vi "Process Methods.vi"(8 "error in (no error)":errorcluster {"code" format="Error %.0f"}, 10 "UIs":refnum<class "GUI Documentation.lvclass">[](array[class]), 11 "VIDoc Printer In":refnum<class "VIDoc Printer.lvclass">) -> (0 "error out":errorcluster {"code" format="Error %.0f"}, 3 "VIDoc Printer Out":refnum<class "VIDoc Printer.lvclass">)   [LabVIEW 2023, in "VIDoc Printer.lvlib" / "VIDoc Printer.lvclass"]
uses:
  VIDoc Printer.lvclass
  VIDoc Printer.lvclass/VIDoc Printer.ctl
  Parsing/GUI Documentation/GUI Documentation.lvclass
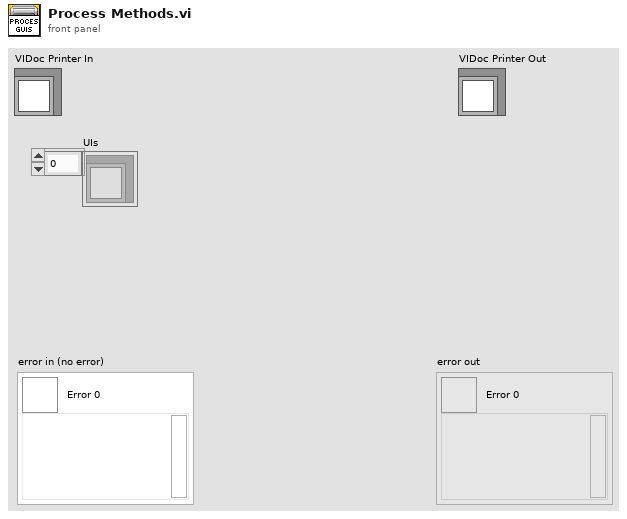
[diagram p1: front panel]
types:
  T1 = typedef "VIDoc Printer.lvlib/VIDoc Printer.lvclass/Process VI Enum.ctl" = enum16{"Header", "Memory", "By Folder", "By Tree", "By List", "Method Details", "FP"}
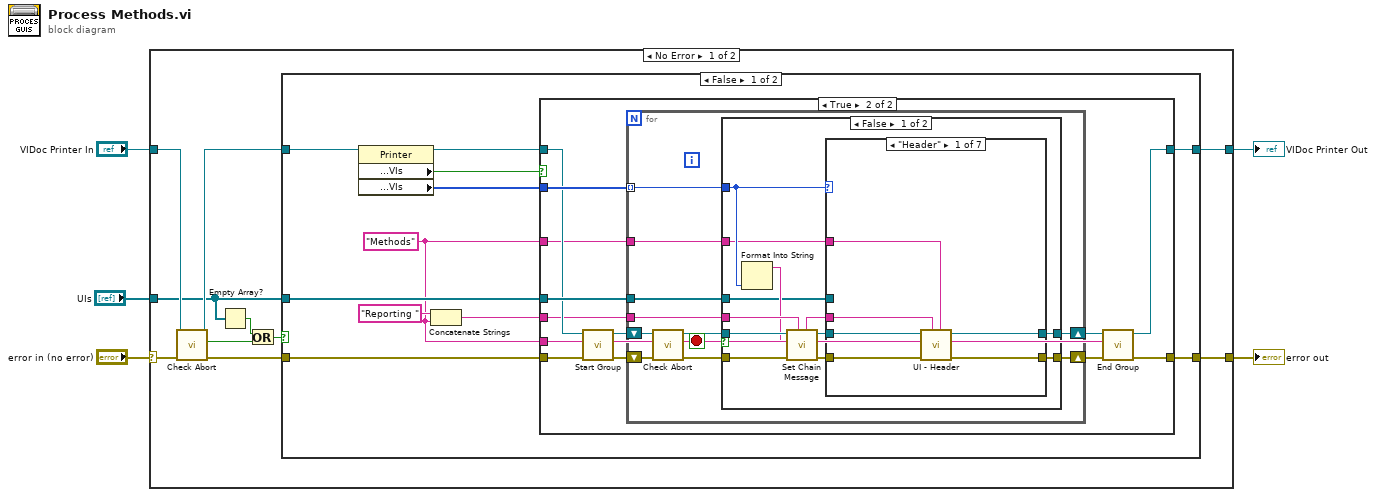
[diagram p0: block diagram]
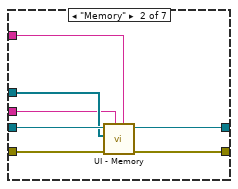
[diagram p3: hidden frame]
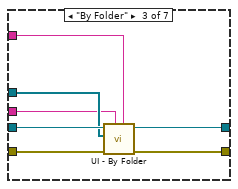
[diagram p4: hidden frame]
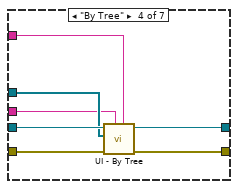
[diagram p5: hidden frame]
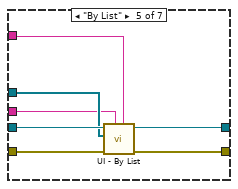
[diagram p6: hidden frame]
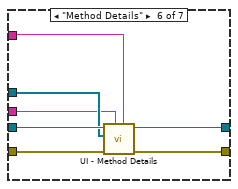
[diagram p7: hidden frame]
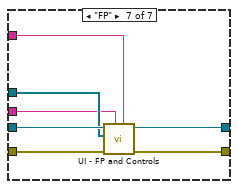
[diagram p8: hidden frame]
diagram:
  n1 = case shown="No Error" "error in (no error)" {
    selector: "error in (no error)" -> [w15 w118]
    tunnel: [w10 w118] -> w4
    tunnel: [w9 w117] -> w2
    tunnel: "VIDoc Printer In" -> [w12 w117]
    tunnel: "UIs" -> [w8 _]
    frame No Error {
      n2 = call "Check Abort.vi"("error in (no error)"=w15, "VIDoc Printer In"=w12) -> ("error out"=w14:errorcluster, "Abort?"=w11:bool, "VIDoc Printer Out"=w13:refnum<class "VIDoc Printer.lvclass">)  [unwired: 7 in]
      n3 = Empty Array?(array=w8) -> (empty?=w6:bool)
      n4 = Or(x=w6, y=w11) -> (x .or. y?=w7:bool)
      n5 = case shown="False" w7 {
        tunnel: w8 -> [w26 _]
        tunnel: w14 -> [w23 w116]
        tunnel: w13 -> [w24 w115]
        tunnel: [w21 w116] -> w10
        tunnel: [w22 w115] -> w9
        frame False {
          w16 = "Methods" ("string")
          n6 = property class="Printer"(reference=w24) -> (reference out=w25:refnum<class "VIDoc Printer.lvclass">, "Properties:Settings:Enabled Sections:VIs"=w18:bool, "Properties:Process Lists:VIs"=w17:T1[])  [unwired: 1 in, 1 out]
          n7 = Concatenate Strings("Reporting " ("string"), w16) -> (w19:string)
          n8 = case shown="True" w18 {
            tunnel: w23 -> [w28 w39]
            tunnel: w19 -> [_ w31]
            tunnel: [w28 w32] -> w21
            tunnel: w26 -> [_ w41]
            tunnel: w25 -> [w27 w36]
            tunnel: [w27 w33] -> w22
            tunnel: w17 -> [_ w40]
            tunnel: w16 -> [_ w30]
            tunnel: w16 -> [_ w29]
            frame False {
            }
            frame True {
              n9 = call-dynamic "Start Group.vi"("error in (no error)"=w39, "Group"=w30, "VIDoc Printer In"=w36) -> ("error out"=w38:errorcluster, "VIDoc Printer Out"=w37:refnum<class "VIDoc Printer.lvclass">)  [unwired: 7 in]
              n10 = for {
                shift-right: [w50] -> w34
                shift-left: w38 -> [w52]
                tunnel: w31 -> [w46]
                tunnel: w41 -> [w45]
                shift-right: [w48] -> w35
                shift-left: w37 -> [w51]
                tunnel: w40 -> [w44] mode=indexing
                tunnel: w29 -> [w42]
                stop <- w43 stop-if-true
                n11 = call "Check Abort.vi"("error in (no error)"=w52, "VIDoc Printer In"=w51) -> ("error out"=w49:errorcluster, "Abort?"=w43:bool, "VIDoc Printer Out"=w47:refnum<class "VIDoc Printer.lvclass">)  [unwired: 7 in]
                n12 = case shown="False" w43 {
                  tunnel: [w64 w114] -> w50
                  tunnel: w49 -> [w61 w114]
                  tunnel: [w63 w113] -> w48
                  tunnel: w47 -> [w59 w113]
                  tunnel: w46 -> [w58 _]
                  tunnel: w45 -> [w55 _]
                  tunnel: w44 -> [w57 _]
                  tunnel: w42 -> [w53 _]
                  frame False {
                    n13 = Format Into String(w57) -> (resulting string=w56:string)  [unwired: 3 in, 1 out]
                    n14 = call "Set Chain Message.vi"("Msg Chain"=w58, "error in (no error)"=w61, "New"=w56, "VIDoc Printer In"=w59) -> ("error out"=w62:errorcluster, "VIDoc Printer Out"=w60:refnum<class "VIDoc Printer.lvclass">, "Msg Chain out"=w54:string)  [unwired: 5 in]
                    n15 = case shown="\"Header\"" w57 {
                      tunnel: w62 -> [w69 w76 w83 w90 w97 w104 w111]
                      tunnel: [w67 w74 w81 w88 w95 w102 w109] -> w64
                      tunnel: w60 -> [w70 w77 w84 w91 w98 w105 w112]
                      tunnel: [w68 w75 w82 w89 w96 w103 w110] -> w63
                      tunnel: w55 -> [_ w73 w80 w87 w94 w101 w108]
                      tunnel: w54 -> [w66 w72 w79 w86 w93 w100 w107]
                      tunnel: w53 -> [w65 w71 w78 w85 w92 w99 w106]
                      frame "Header" {
                        n16 = call-dynamic "UI - Header.vi"("Term (Methods)"=w65, "Msg Chain"=w66, "error in"=w69, "VIDoc Printer In"=w70) -> ("error out"=w67:errorcluster, "VIDoc Printer Out"=w68:refnum<class "VIDoc Printer.lvclass">)  [unwired: 6 in]
                      }
                      frame "Memory" {
                        n17 = call-dynamic "UI - Memory.vi"("Term (Methods)"=w71, "Msg Chain"=w72, "error in (no error)"=w76, "UI Docs"=w73, "VIDoc Printer In"=w77) -> ("error out"=w74:errorcluster, "VIDoc Printer Out"=w75:refnum<class "VIDoc Printer.lvclass">)  [unwired: 5 in]
                      }
                      frame "By Folder" {
                        n18 = call-dynamic "UI - By Folder.vi"("Term (Methods)"=w78, "Msg Chain"=w79, "error in (no error)"=w83, "UI Docs"=w80, "VIDoc Printer In"=w84) -> ("error out"=w81:errorcluster, "VIDoc Printer Out"=w82:refnum<class "VIDoc Printer.lvclass">)  [unwired: 5 in]
                      }
                      frame "By Tree" {
                        n19 = call-dynamic "UI - By Tree.vi"("Term (Methods)"=w85, "Msg Chain"=w86, "error in (no error)"=w90, "UI Docs"=w87, "VIDoc Printer In"=w91) -> ("error out"=w88:errorcluster, "VIDoc Printer Out"=w89:refnum<class "VIDoc Printer.lvclass">)  [unwired: 5 in]
                      }
                      frame "By List" {
                        n20 = call-dynamic "UI - By List.vi"("Term (Methods)"=w92, "Msg Chain"=w93, "error in (no error)"=w97, "UI Docs"=w94, "VIDoc Printer In"=w98) -> ("error out"=w95:errorcluster, "VIDoc Printer Out"=w96:refnum<class "VIDoc Printer.lvclass">)  [unwired: 5 in]
                      }
                      frame "Method Details" {
                        n21 = call-dynamic "UI - Method Details.vi"("Term (Methods)"=w99, "Msg Chain"=w100, "error in (no error)"=w104, "UI Docs"=w101, "VIDoc Printer In"=w105) -> ("error out"=w102:errorcluster, "VIDoc Printer Out"=w103:refnum<class "VIDoc Printer.lvclass">)  [unwired: 5 in]
                      }
                      frame "FP" {
                        n22 = call-dynamic "UI - FP and Controls.vi"("Term (Methods)"=w106, "Msg Chain"=w107, "error in (no error)"=w111, "UI Docs"=w108, "VIDoc Printer In"=w112) -> ("error out"=w109:errorcluster, "VIDoc Printer Out"=w110:refnum<class "VIDoc Printer.lvclass">)  [unwired: 5 in]
                      }
                    }
                  }
                  frame True {
                  }
                }
              }
              n23 = call-dynamic "End Group.vi"("error in (no error)"=w34, "Group"=w30, "VIDoc Printer In"=w35) -> ("error out"=w32:errorcluster, "VIDoc Printer Out"=w33:refnum<class "VIDoc Printer.lvclass">)  [unwired: 7 in]
            }
          }
        }
        frame True {
        }
      }
    }
    frame Error {
    }
  }
  "error out" <- w4
  "VIDoc Printer Out" <- w2
